vi "Get CI Frequency Terminal.vi"(0 "Task Name":refnum<k21>, 5 "channel":string) -> (4 "CI.Freq.Term":tag)   [LabVIEW 2021, in "NIDAQmxMeasurement.lvlib"]
doc: "Gets the Counter Input Frequency Terminal resource from task name and channel name."
uses:
  NIDAQmxMeasurement.lvlib
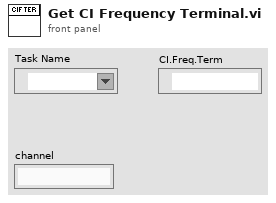
[diagram p1: front panel]
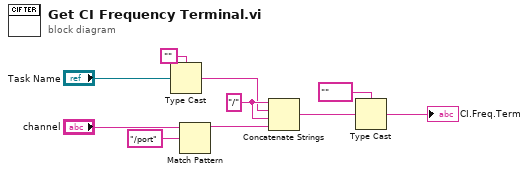
[diagram p0: block diagram]
diagram:
  w6 = "/" ("string")
  n1 = Type Cast(type="", x="Task Name") -> (*(type *) &x=w1:string)
  n2 = Match Pattern(string="channel", regular expression="/port") -> (before substring=w8:string)  [unwired: 1 in, 3 out]
  n3 = Concatenate Strings(w6, w1, w6, w8) -> (w9:string)
  n4 = Type Cast(type=tag "" ("CI.Freq.Term"), x=w9) -> (*(type *) &x=→"CI.Freq.Term":tag)
